vi "checkM9347driver.vi"(8 "error in (no error)":errorcluster) -> (0 "error out":errorcluster, 3 "Checkbox":bool)   [LabVIEW 2023]
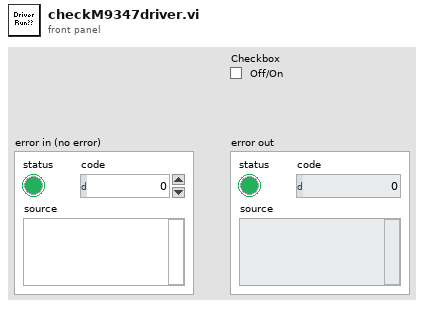
[diagram p1: front panel]
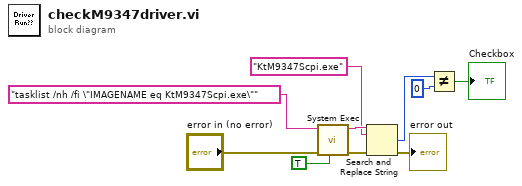
[diagram p0: block diagram]
diagram:
  n1 = call <vilib>:"System Exec.vi"("run minimized? (F)"=TRUE, "error in (no error)"="error in (no error)", "command line"="tasklist /nh /fi \"IMAGENAME eq KtM9347Scpi.exe\"") -> ("error out"=w9:errorcluster, "standard output"=w5:string)  [unwired: 5 in, 2 out]
  n2 = Search and Replace String(input string=w5, search string="KtM9347Scpi.exe", error in=w9) -> (number of replacements=w6:i32, error out=→"error out":errorcluster)  [unwired: 5 in, 2 out]
  n3 = Not Equal?(x=w6, y=0) -> (x != y?=→"Checkbox":bool)
